vi "Link UI.vi"(8 "error in (no error)":errorcluster, 10 "<2> 2":string, 11 "<2>":string) -> (0 "error out":errorcluster)   [LabVIEW 2020, in "CSM-FileSync.lvlib"]
uses:
  CSM-FileSync.lvlib
  <userlib>/_NEVSTOP/Communicable State Machine(CSM)/_Polymophic/CSM - Replace Marks in Messages.vi
  <userlib>/_NEVSTOP/Communicable State Machine(CSM)/Communicable State Machine.lvlib
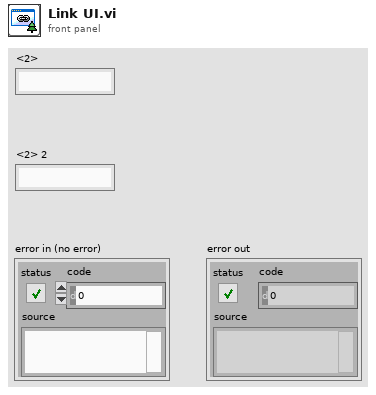
[diagram p1: front panel]
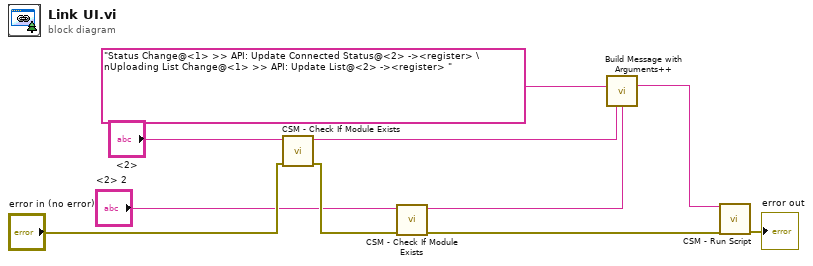
[diagram p0: block diagram]
diagram:
  n1 = call <userlib>:"CSM - Check If Module Exists.vi"("Error In"="error in (no error)", "CSM Name"="<2>") -> ("error out"=w8:errorcluster, "CSM Name (Dup)"=w7:string)  [unwired: 7 in, 1 out]
  n2 = call <userlib>:"CSM - Check If Module Exists.vi"("Error In"=w8, "CSM Name"="<2> 2") -> ("error out"=w10:errorcluster, "CSM Name (Dup)"=w6:string)  [unwired: 7 in, 1 out]
  n3 = call-poly <userlib>:"Build Message with Arguments++.vi"("States With Replace Token"="Status Change@<1> >> API: Update Connected Status@<2> -><register> \nUploading List Change@<1> >> API: Update List@<2> -><register> " ("CSM Scripts"), "<1>"=w7, "<2>"=w6) -> ("States"=w2:string)  [unwired: 12 in]
  n4 = call <userlib>:"CSM - Run Script.vi"("CSM Scripts"=w2, "error in (no error)"=w10) -> ("error out"=→"error out":errorcluster)  [unwired: 11 in, 2 out]
